vi "PR.vi"(8 "error in (no error)":errorcluster, 9 "Target Position":i64, 10 "Axis Number":i32, 11 "Agilis in":T1) -> (0 "error out":errorcluster, 3 "Agilis out":T1)   [LabVIEW 2016, in "Drivers.lvlib" / "Agilis.lvlib"]
doc: "Starts a relative move of steps with step amplitude defined by SU."
uses:
  Agilis.lvlib
  AgilisCmdLib Refnum.ctl
  D:/Trace Grabber/Drivers/Agilis/AgilisCmdLib.dll
  AgilisCmdLib.dll
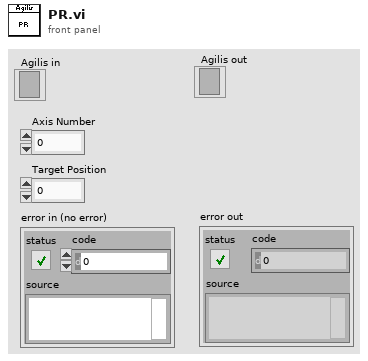
[diagram p1: front panel]
types:
  T1 = typedef "Drivers.lvlib/Agilis.lvlib/AgilisCmdLib Refnum.ctl" = refnum<k24>
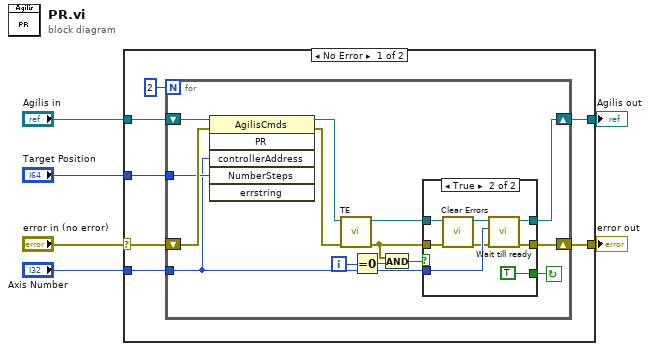
[diagram p0: block diagram]
diagram:
  n1 = case shown="No Error" "error in (no error)" {
    selector: "error in (no error)" -> [w12 w38]
    tunnel: "Agilis in" -> [w13 w37]
    tunnel: [w8 w37] -> w4
    tunnel: [w9 w38] -> w3
    tunnel: "Axis Number" -> [w11 _]
    tunnel: "Target Position" -> [w10 _]
    frame No Error {
      n2 = for {
        N: 2 -> [_]
        tunnel: w11 -> [w19]
        tunnel: w10 -> [w25]
        shift-right: [w20] -> w8
        shift-left: w13 -> [w27]
        shift-right: [w22] -> w9
        shift-left: w12 -> [w26]
        i -> [w15]
        stop <- w18 continue-if-true
        n3 = invoke class="AgilisCmds" method="PR"(reference=w27, error in=w26, "controllerAddress"=w19, "NumberSteps"=w25) -> (reference out=w23:T1, error out=w24:errorcluster)  [unwired: 2 in, 4 out]
        n4 = call "TE.vi"("error in (no error)"=w24, "Agilis in"=w23) -> ("error out"=w16:errorcluster, "Agilis out"=w21:T1)  [unwired: 8 in]
        n5 = Equal To 0?(x=w15) -> (x = 0?=w14:bool)
        n6 = And(x=w16, y=w14) -> (x .and. y?=w17:bool)
        n7 = case shown="True" w17 {
          tunnel: [w28 w36] -> w22
          tunnel: w21 -> [w29 w35]
          tunnel: [w29 w34] -> w20
          tunnel: w19 -> [_ w33]
          tunnel: [_ TRUE] -> w18
          tunnel: w16 -> [w28 w31]
          frame False {
          }
          frame True {
            n8 = call <vilib>:"Clear Errors.vi"("error in (no error)"=w31) -> ("error out"=w30:errorcluster)  [unwired: 5 in, 1 out]
            n9 = call "Wait till ready.vi"("error in (no error)"=w30, "Axis Number"=w33, ".NET Refnum in"=w35) -> ("error out"=w36:errorcluster, ".NET Refnum out"=w34:T1)  [unwired: 7 in]
          }
        }
      }
    }
    frame Error {
    }
  }
  "Agilis out" <- w4
  "error out" <- w3
